vi "Plot add row if filled.vi"(8 "error in (no error)":errorcluster, 10 "top array":T1[](array[typedef]), 11 "Refs":T2) -> (0 "error out":errorcluster, 3 "Row added?":bool)   [LabVIEW 2021, in "RocketPlot.lvlib"]
uses:
  RocketPlot.lvlib
  TypeDefs/Plot UI references.ctl
  Classes/RocketPlotHandle/RocketPlotHandle.lvclass
  <userlib>/bjustice/TipStripOOPanel/Classes/TipPanelHandle/TipPanelHandle.lvclass
  TypeDefs/Plot top row.ctl
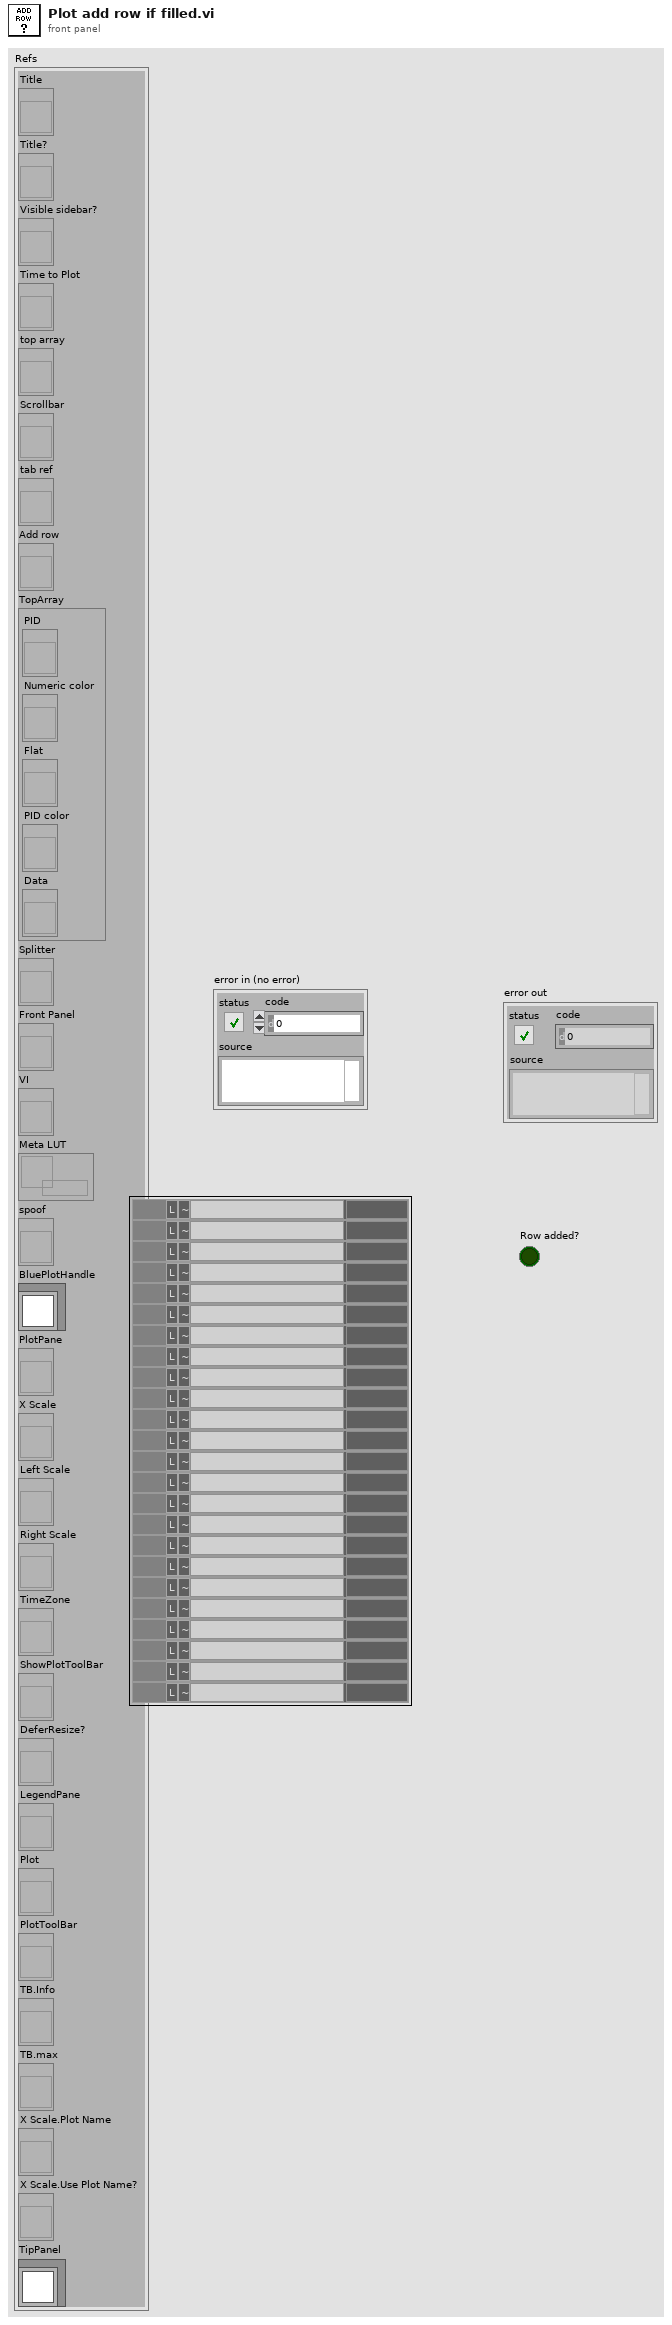
[diagram p1: front panel]
types:
  T1 = typedef "RocketPlot.lvlib/Plot top row.ctl" = cluster{"PID":string, "index":i32, "PID color":u32, "right axis?":bool, "Flatline?":bool, "Numeric color":u32, "Data":string, "Flat":string}
  T2 = typedef "RocketPlot.lvlib/Plot UI references.ctl" = cluster{"Title":refnum<vi>, "Title?":refnum<vi>, "Visible sidebar?":refnum<vi>, "Time to Plot":refnum<vi>, "top array":refnum<vi>, "Scrollbar":refnum<vi>, "tab ref":refnum<vi>, "Add row":refnum<vi>, "TopArray":cluster{"PID":refnum<vi>, "Numeric color":refnum<vi>, "Flat":refnum<vi>, "PID color":refnum<vi>, "Data":refnum<vi>}, "Splitter":refnum<vi>, "Front Panel":refnum<vi>, "VI":refnum<vi>, "Meta LUT":refnum<data-value>, "spoof":refnum<vi>, "BluePlotHandle":refnum<class "RocketPlotHandle.lvclass">, "PlotPane":refnum<vi>, "X Scale":refnum<vi>, "Left Scale":refnum<vi>, "Right Scale":refnum<vi>, "TimeZone":refnum<vi>, "ShowPlotToolBar":refnum<vi>, "DeferResize?":refnum<vi>, "LegendPane":refnum<vi>, "Plot":refnum<vi>, "PlotToolBar":refnum<vi>, "TB.Info":refnum<vi>, "TB.max":refnum<vi>, "X Scale.Plot Name":refnum<vi>, "X Scale.Use Plot Name?":refnum<vi>, "TipPanel":refnum<class "TipPanelHandle.lvclass">}
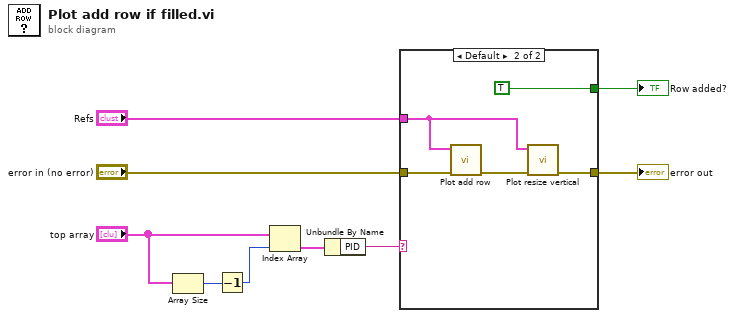
[diagram p0: block diagram]
diagram:
  n1 = Array Size(array="top array") -> (size(s)=w8:i32)
  n2 = Decrement(x=w8) -> (x-1=w7:i32)
  n3 = Index Array(array="top array", index=w7) -> (element=w5:T1)
  n4 = Unbundle By Name(w5) -> ("PID"=w4:string)
  n5 = case shown="Default" w4 {
    tunnel: "Refs" -> [_ w11]
    tunnel: "error in (no error)" -> [w10 w14]
    tunnel: [w10 w13] -> w2
    tunnel: [_ TRUE] -> w1
    frame "" {
    }
    frame Default {
      n6 = call "Plot add row.vi"("error in (no error)"=w14, "Refs"=w11) -> ("error out"=w15:errorcluster)  [unwired: 9 in]
      n7 = call "Plot resize vertical.vi"("error in (no error)"=w15, "Refs"=w11) -> ("error out"=w13:errorcluster)  [unwired: 7 in, 2 out]
    }
  }
  "error out" <- w2
  "Row added?" <- w1
